vi "Test des thermistances.vi"() -> ()   [LabVIEW 2020]
uses:
  <vilib>/Waveform/WDTFileIO.llb/Export Waveform To Spreadsheet File.vi
  <vilib>/Waveform/WDTOps.llb/WDT Append Waveforms DBL.vi
panel:
  out "Graphique de la thermistance":waveform(dbl)(graph)
  in  "stop":bool
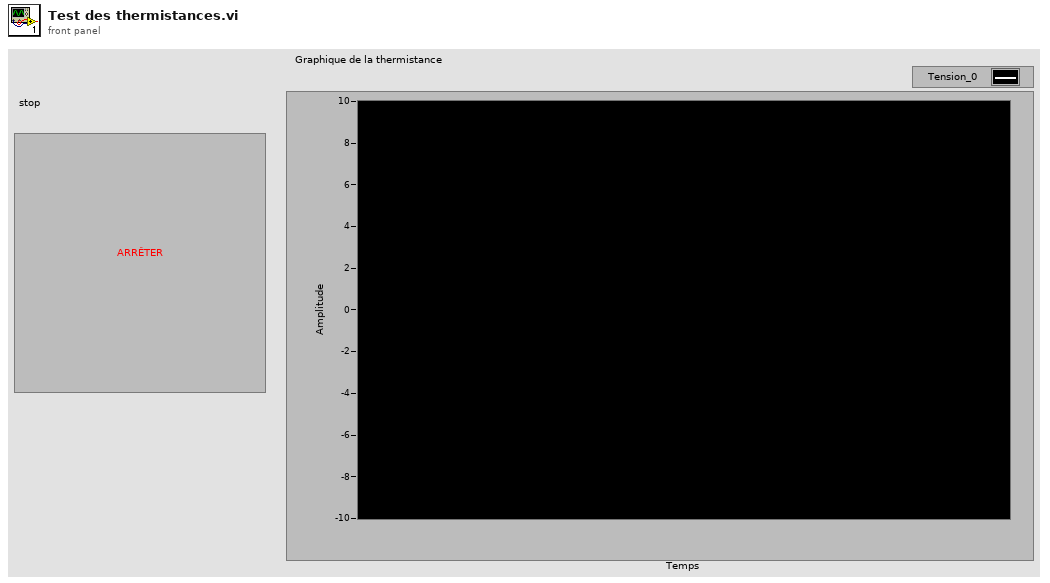
[diagram p1: front panel]
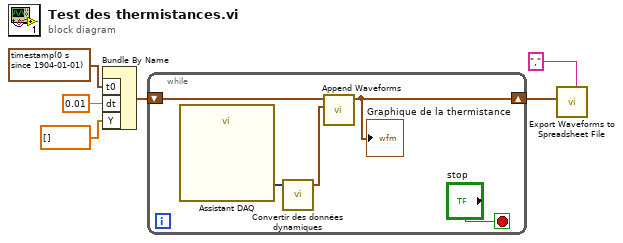
[diagram p0: block diagram]
diagram:
  n1 = Bundle By Name("t0"=timestamp(0 s since 1904-01-01), "dt"=0.01, "Y"=dbl[] []) -> (w3:waveform(dbl))  [unwired: 1 in]
  n2 = while {
    shift-right: [w7] -> w2
    shift-left: w3 -> [w9]
    stop <- "stop" stop-if-true
    n3 = call "Assistant DAQ"() -> ("data"=w10:dynamicdata)  [unwired: 17 in, 2 out]
    n4 = call "Convertir des données dynamiques"("Dynamic Data Type"=w10) -> ("Waveform"=w8:waveform(dbl))  [unwired: 3 in]
    n5 = call-poly <vilib>:"Append Waveforms.vi"("waveform B"=w8, "waveform A"=w9) -> ("waveform out"=w7:waveform(dbl))  [unwired: 8 in, 1 out]
    "Graphique de la thermistance" <- w7
  }
  n6 = call-poly <vilib>:"Export Waveforms to Spreadsheet File.vi"("delimiter (Tab)"=",", "waveform"=w2) -> ()  [unwired: 8 in, 2 out]
